vi "timekeeper time rate adjust valid (g).vi"() -> ()   [LabVIEW 2011, in "EPS_Timekeeper.lvlib"]
uses:
  <vilib>/addons/Electrical Power/Example Support/PMU/Time Keeper/EPS_Timekeeper.lvlib
panel:
  in  "time rate adjust change (g)":bool
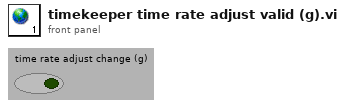
[diagram p1: front panel]
diagram:
